vi "HandshakeResponse.vi"(4 "error in (no error)":errorcluster, 7 "Sec-WebSocket-Key":string) -> (0 "error out":errorcluster, 3 "Response Headers":string)   [LabVIEW 2015, in "WebSockets.lvlib"]
doc: "Creates the HTTP handshaking response.\nWebSockets API 1.3.0.13\nSam Sharp - Intelligent Energy\nCopyright (c) 2015, Intelligent Energy"
uses:
  WebSockets.lvlib
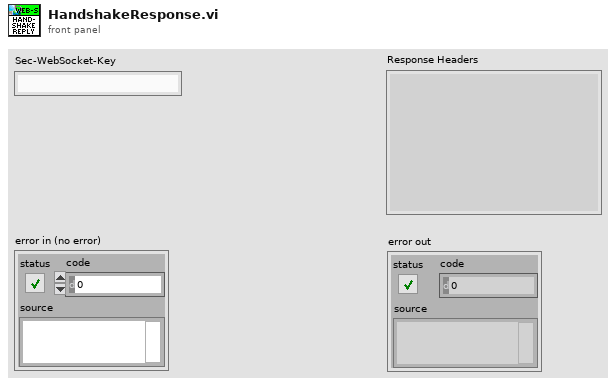
[diagram p1: front panel]
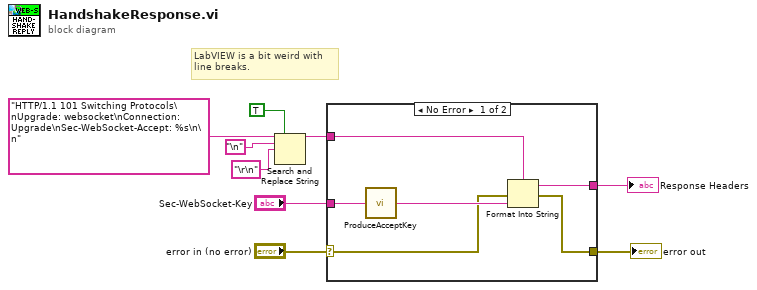
[diagram p0: block diagram]
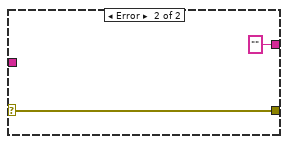
[diagram p2: hidden frame]
diagram:
  # "LabVIEW is a bit weird with line breaks."
  n1 = Search and Replace String(replace all?=TRUE ("replace all? (F)"), input string="HTTP/1.1 101 Switching Protocols\nUpgrade: websocket\nConnection: Upgrade\nSec-WebSocket-Accept: %s\n\n" ("format string"), search string="\n", replace string="\r\n" ("search string/char (-)")) -> (result string=w3:string)  [unwired: 4 in, 3 out]
  n2 = case shown="No Error" "error in (no error)" {
    selector: "error in (no error)" -> [w10 w17]
    tunnel: "Sec-WebSocket-Key" -> [w15 _]
    tunnel: w3 -> [w14 _]
    tunnel: [w12 ""] -> w8
    tunnel: [w11 w17] -> w6
    frame No Error {
      n3 = call "ProduceAcceptKey.vi"("Sec-WebSocket-Key"=w15) -> ("Sec-WebSocket-Accept"=w13:string)
      n4 = Format Into String(format string=w14, error in=w10, w13) -> (resulting string=w12:string, error out=w11:errorcluster)  [unwired: 1 in]
    }
    frame Error {
    }
  }
  "Response Headers" <- w8
  "error out" <- w6
